vi "Write to File.vi"(7 "Column Header":string[][](array[string])=[["Time (Rel)", "Time (Abs)", "Pump Elapsed Time", "PS Voltage", "Controller Cmd", "Pump/Ctrl Voltage", "Pump Current", "Controller Current", "Target Speed", "Pump Speed", "Press/Flow Cmd", "Pump Pressure", "Pump Flow", "Tank 1 Temp Cmd", "Tank 1 Temp", "Tank 2 Temp Cmd", "Tank 2 Temp"], ["Hours", "Seconds", "Seconds", "Volts", "%", "Volts", "Amps", "Amps", "RPM", "RPM", "", "kPA", "LPH", "degC", "degC", "degC", "degC"]], 9 "Filename":string, 10 "Data":string[](array[string]), 11 "Path":path) -> ()   [LabVIEW 2013]
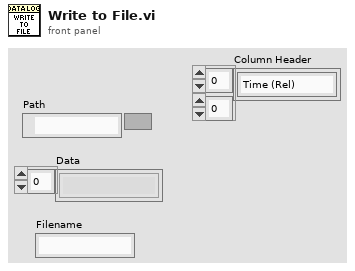
[diagram p1: front panel]
types:
  T1 = enum16{"open", "replace", "create", "open or create", "replace or create", "replace or create with confirmation"}
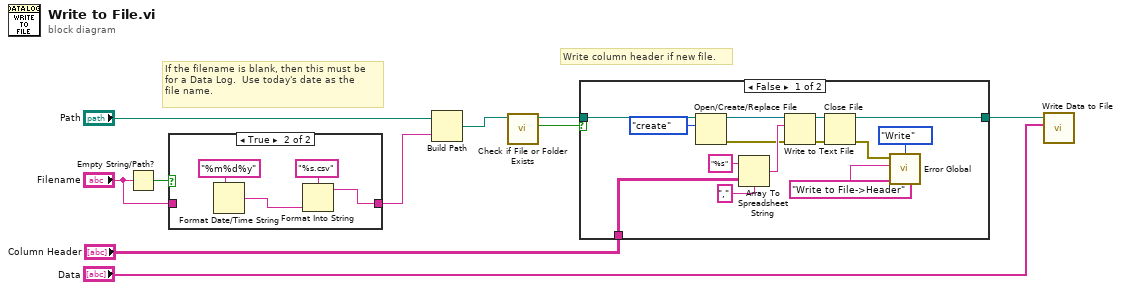
[diagram p0: block diagram]
diagram:
  # "If the filename is blank, then this must be\nfor a Data Log.  Use today's date as the\nfile name."
  # "Write column header if new file."
  n1 = Empty String/Path?(string/path="Filename") -> (empty?=w6:bool)
  n2 = case shown="True" w6 {
    tunnel: "Filename" -> [w11 _]
    tunnel: [w11 w12] -> w4
    frame False {
    }
    frame True {
      n3 = Format Date/Time String(time format string (%c)="%m%d%y") -> (date/time string=w14:string)  [unwired: 2 in]
      n4 = Format Into String(format string="%s.csv", w14) -> (resulting string=w12:string)  [unwired: 2 in, 1 out]
    }
  }
  n5 = Build Path(base path="Path", name or relative path=w4) -> (appended path=w7:path)
  n6 = call <vilib>:"Check if File or Folder Exists.vi"("path"=w7) -> ("file or folder exists?"=w10:bool, "dup path"=w3:path)  [unwired: 8 in, 1 out]
  n7 = case shown="False" w10 {
    tunnel: w3 -> [w20 w30]
    tunnel: "Column Header" -> [w16 _]
    tunnel: [w19 w30] -> w2
    frame False {
      n8 = Open/Create/Replace File(file path (use dialog)=w20, operation (0:open)=T1."create") -> (refnum out=w18:refnum<file>, error out=w17:errorcluster)  [unwired: 4 in, 1 out]
      n9 = Array To Spreadsheet String(delimiter (Tab)=",", array=w16, 3:"%s" ("format string")) -> (spreadsheet string=w26:string)
      n10 = Write to Text File(file (use dialog)=w18, text=w26, error in=w17) -> (refnum out=w22:refnum<file>, error out=w21:errorcluster)  [unwired: 1 in, 1 out]
      n11 = Close File(refnum=w22, error in=w21) -> (path=w19:path, error out=w28:errorcluster)
      n12 = call "Error Global.vi"("Mode"=enum16{"Read", "Write", "Clear Error"}."Write", "Error In"=w28, "Location In"="Write to File->Header" ("delimiter (Tab)")) -> ()  [unwired: 6 in, 2 out]
    }
    frame True {
    }
  }
  n13 = call "Write Data to File.vi"("Data"="Data", "File Path"=w2) -> ()  [unwired: 10 in]
